vi "수신2.vi"() -> ()   [LabVIEW 2023]
panel:
  out "Waveform Graph":dbl[](graph)
  in  "stop":bool
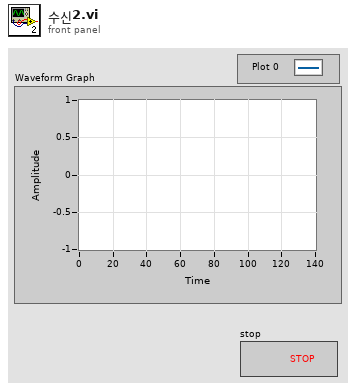
[diagram p1: front panel]
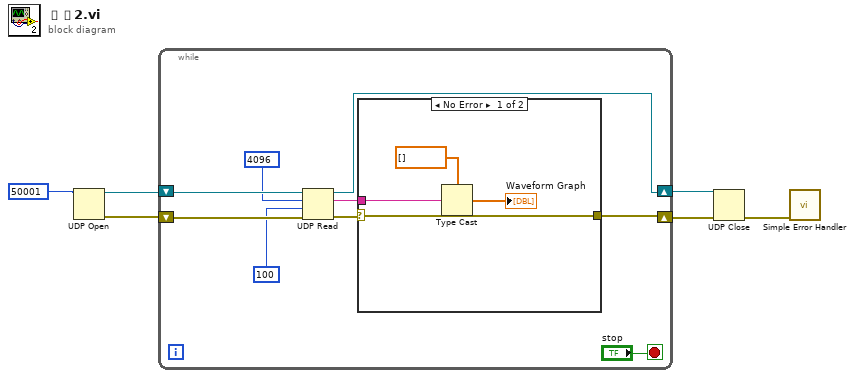
[diagram p0: block diagram]
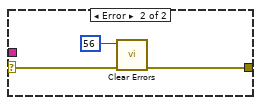
[diagram p2: hidden frame]
diagram:
  n1 = UDP Open(11:u16 50001 ("port")) -> (port=w6:refnum<k16>, 0:w5:errorcluster)  [unwired: 4 in, 1 out]
  n2 = while {
    shift-right: [w14] -> w4
    shift-left: w5 -> [w10]
    shift-right: [w13] -> w2
    shift-left: w6 -> [w12]
    stop <- "stop" stop-if-true
    n3 = UDP Read(connection ID=w12, max size (548)=4096, timeout ms (25000)=100, 8:w10) -> (data out=w11:string, error out=w15:errorcluster, 3:w13:refnum<k16>)  [unwired: 2 out]
    n4 = case shown="No Error" w15 {
      selector: w15 -> [w19 w22]
      tunnel: [w19 w21] -> w14
      tunnel: w11 -> [w18 _]
      frame No Error {
        n5 = Type Cast(type=dbl[] [] ("Waveform Graph"), x=w18) -> (*(type *) &x=→"Waveform Graph":dbl[])
      }
      frame Error {
        n6 = call <vilib>:"Clear Errors.vi"("error in (no error)"=w22, "specific error code to clear (0: all)"=56) -> ("error out"=w21:errorcluster)  [unwired: 4 in, 1 out]
      }
    }
  }
  n7 = UDP Close(connection ID=w2, 8:w4) -> (error out=w3:errorcluster)  [unwired: 1 out]
  n8 = call <vilib>:"Simple Error Handler.vi"("error in (no error)"=w3) -> ()  [unwired: 4 in, 5 out]
